vi "Configure Terminals.vi"(11 "State in":T2) -> (2 "cancelled?":bool, 3 "State out":T2)   [LabVIEW 2015]
uses:
  State.ctl
  Get Object Parameters/Parameter.ctl
  Set Object Parameters.xnode
  Shared/Shared.lvlib
panel:
  in  "Terminals":T1[](array[typedef])
  in  "Cancel_Button":bool
  in  "OK_Button":bool
  # "Parameter Name"
  # "JSON Type"
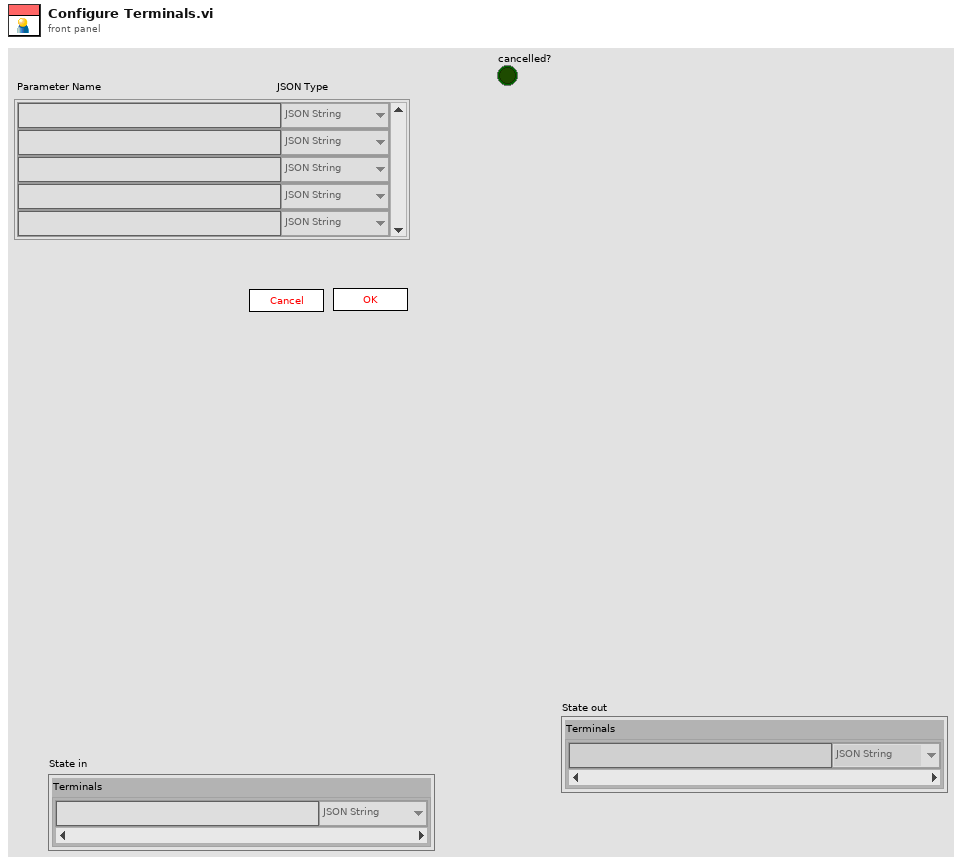
[diagram p1: front panel]
types:
  T1 = typedef "LVJSON.lvlib/Shared.lvlib/Parameter.ctl" = cluster{"Parameter Name":string, "JSON Type":enum16{"JSON String", "JSON Numeric", "JSON Boolean", "JSON", "JSON Object", "JSON Array", "String Value", "Numeric Value", "Boolean Value"}}
  T2 = typedef "LVJSON.lvlib/Set Object Parameters.xnode/State.ctl" = cluster{"Terminals":T1[]}
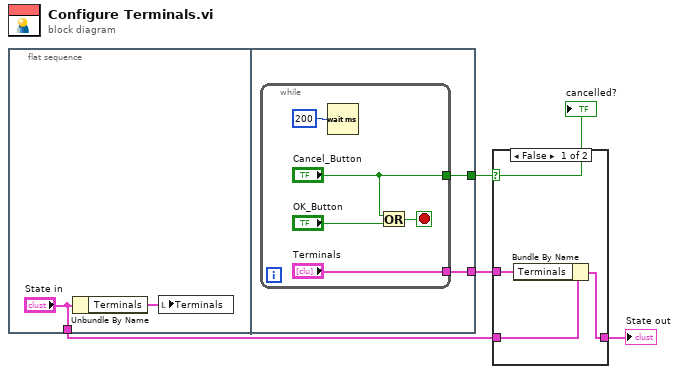
[diagram p0: block diagram]
diagram:
  n1 = flat-sequence {
    tunnel: ["State in"] -> w4
    tunnel: [w8] -> w2
    tunnel: [w7] -> w1
    frame #0 {
      n2 = Unbundle By Name("State in") -> ("Terminals"=w5:T1[])
      n3 = local write "Terminals"(w5) -> ()
    }
    frame #1 {
      n4 = while {
        tunnel: ["Terminals"] -> w8
        tunnel: ["Cancel_Button"] -> w7
        stop <- w10 stop-if-true
        n5 = Wait (ms)(milliseconds to wait=u32 200) -> ()  [unwired: 1 out]
        n6 = Or(x="Cancel_Button", y="OK_Button") -> (x .or. y?=w10:bool)
      }
    }
  }
  n7 = case shown="False" w1 {
    tunnel: w4 -> [w16 w17]
    tunnel: [w15 w17] -> w3
    tunnel: w2 -> [w14 _]
    frame False {
      n8 = Bundle By Name(cluster=w16, "Terminals"=w14) -> (w15:T2)
    }
    frame True {
    }
  }
  "State out" <- w3
  "cancelled?" <- w1
